vi "LEP_RV_SetupBuildFolder.vi"(2 "error in (no error)":errorcluster, 4 "Build Path":path) -> (0 "error out":errorcluster, 1 "Status":T1(ring)=enum."EmptyTopLevelVIPath")   [LabVIEW 2011]
doc: "Creates the <B>Build Path</B> directory."
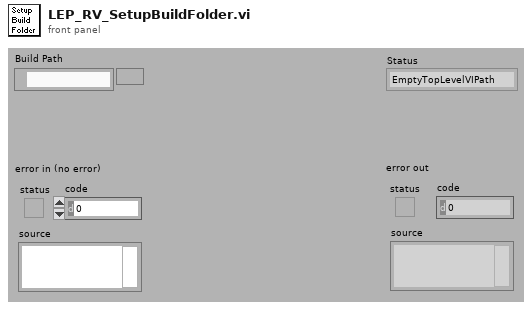
[diagram p1: front panel]
types:
  T1 = enum16{"NoErr", "TopLevelVIErr", "EmptyTopLevelVIPath", "CGenErr", "CpySuppFilesErr", "ProjectInfoErr", "NoTopLevelVIErr", "CreateBuildFolderErr", "EmptyBuildFolderErr", "LoadConfigErr", "BildToolsErr", "CompileErr", "LinkError", "DebugInfoErr", "NotFoundErr", "AccessErr", "ExecErr", "UnknownErr"}
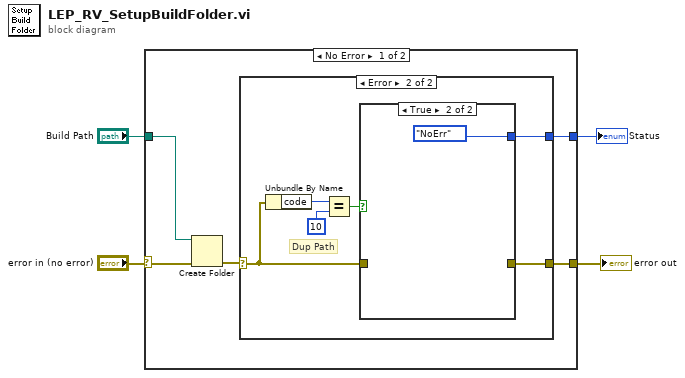
[diagram p0: block diagram]
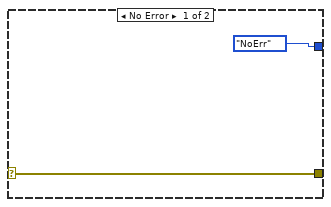
[diagram p2: hidden frame]
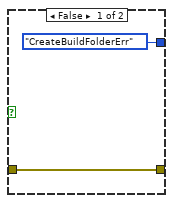
[diagram p3: hidden frame]
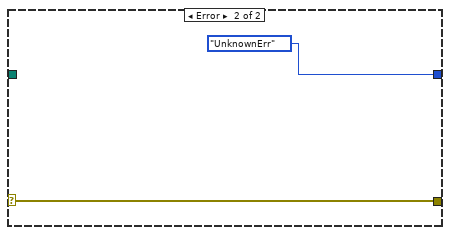
[diagram p4: hidden frame]
diagram:
  n1 = case shown="No Error" "error in (no error)" {
    selector: "error in (no error)" -> [w7 w22]
    tunnel: [w9 T1."UnknownErr" ("Errors")] -> w1
    tunnel: [w8 w22] -> w3
    tunnel: "Build Path" -> [w5 _]
    frame No Error {
      n2 = Create Folder(path (use dialog)=w5, error in=w7) -> (error out=w6:errorcluster)  [unwired: 1 in, 2 out]
      n3 = case shown="Error" w6 {
        selector: w6 -> [w11 w14]
        tunnel: [w11 w13] -> w8
        tunnel: [T1."NoErr" ("Errors") w12] -> w9
        frame No Error {
        }
        frame Error {
          # "Dup Path"
          n4 = Unbundle By Name(w14) -> ("code"=w17:i32)
          n5 = Equal?(x=w17, y=10) -> (x = y?=w15:bool)
          n6 = case shown="True" w15 {
            tunnel: w14 -> [w19 _]
            tunnel: [w19 _] -> w13
            tunnel: [T1."CreateBuildFolderErr" ("Errors") T1."NoErr" ("Errors")] -> w12
            frame False {
            }
            frame True {
            }
          }
        }
      }
    }
    frame Error {
    }
  }
  "error out" <- w3
  "Status" <- w1
